vi "Get Disabled Items.vi"(8 "error in (no error)":errorcluster, 11 "Listbox or Tree":refnum<vi>) -> (0 "error out":errorcluster, 3 "Disabled Items":i32[](array[numeric]))   [LabVIEW 2011]
doc: "This VI gets the disabled indexes for a Listbox, MCLB, or Tree control.\n-------------\nBrian Hoover (hooovahh)"
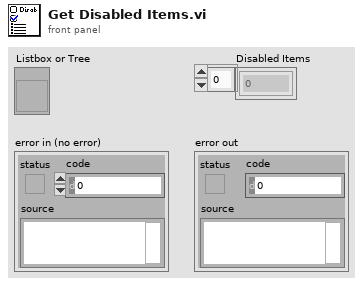
[diagram p1: front panel]
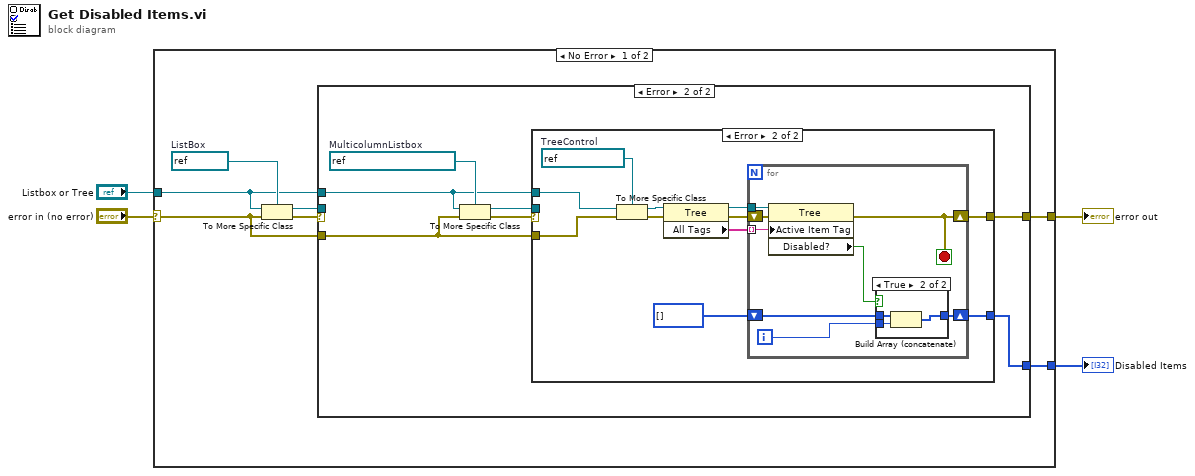
[diagram p0: block diagram]
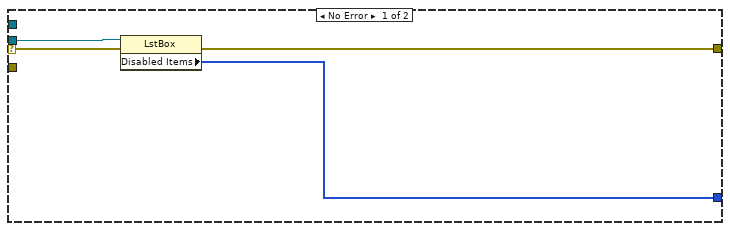
[diagram p2: hidden frame]
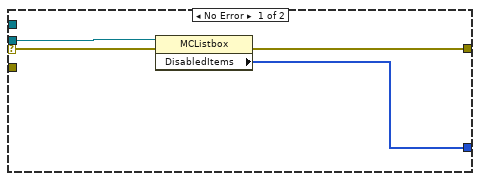
[diagram p3: hidden frame]
diagram:
  n1 = case shown="No Error" "error in (no error)" {
    selector: "error in (no error)" -> [w7 w50]
    tunnel: [w11 w50] -> w4
    tunnel: "Listbox or Tree" -> [w6 _]
    tunnel: [w5 _] -> w1
    frame No Error {
      w8 = refnum<vi> refnum  # ListBox
      n2 = To More Specific Class(target class=w8, reference=w6, error in=w7) -> (specific class reference=w10:refnum<vi>, error out=w9:errorcluster)
      n3 = case shown="Error" w9 {
        selector: w9 -> [w14 _]
        tunnel: w10 -> [w15 _]
        tunnel: w7 -> [_ w17]
        tunnel: [w13 w19] -> w11
        tunnel: w6 -> [_ w16]
        tunnel: [w12 w18] -> w5
        frame No Error {
          n4 = property class="LstBox"(reference=w15, error in=w14) -> (error out=w13:errorcluster, "Disabled Items"=w12:i32[])  [unwired: 1 out]
        }
        frame Error {
          w22 = refnum<vi> refnum  # MulticolumnListbox
          n5 = To More Specific Class(target class=w22, reference=w16, error in=w17) -> (specific class reference=w21:refnum<vi>, error out=w20:errorcluster)
          n6 = case shown="Error" w20 {
            selector: w20 -> [w24 _]
            tunnel: [w26 w36] -> w19
            tunnel: w21 -> [w25 _]
            tunnel: [w23 w35] -> w18
            tunnel: w17 -> [_ w34]
            tunnel: w16 -> [_ w33]
            frame No Error {
              n7 = property class="MCListbox"(reference=w25, error in=w24) -> (error out=w26:errorcluster, "DisabledItems"=w23:i32[])  [unwired: 1 out]
            }
            frame Error {
              w37 = refnum<vi> refnum  # TreeControl
              n8 = To More Specific Class(target class=w37, reference=w33, error in=w34) -> (specific class reference=w29:refnum<vi>, error out=w32:errorcluster)
              n9 = property class="Tree"(reference=w29, error in=w32) -> (reference out=w28:refnum<vi>, error out=w30:errorcluster, "All Tags"=w31:string[])
              n10 = for {
                tunnel: w28 -> [w45]
                tunnel: w31 -> [w43] mode=indexing
                shift-right: [w42] -> w36
                shift-left: w30 -> [w44]
                shift-right: [w38] -> w35
                shift-left: i32[] [] ("Array") -> [w39]
                i -> [w41]
                stop <- w42 stop-if-true
                n11 = property class="Tree"(reference=w45, error in=w44, "Active Item Tag"=w43) -> (error out=w42:errorcluster, "Disabled?"=w40:bool)  [unwired: 1 out]
                n12 = case shown="True" w40 {
                  tunnel: w39 -> [w46 w48]
                  tunnel: w41 -> [_ w47]
                  tunnel: [w46 w49] -> w38
                  frame False {
                  }
                  frame True {
                    n13 = Build Array (concatenate)(w48, w47) -> (w49:i32[])
                  }
                }
              }
            }
          }
        }
      }
    }
    frame Error {
    }
  }
  "error out" <- w4
  "Disabled Items" <- w1
